vi "Insight_RW_Sweep_Profile.vi"(6 "String":string, 7 "Edge Roll-off (dB)":dbl=10.0 min=0.0 max=0.0, 8 "error in (no error)":errorcluster, 9 "Mode (Read / Write)":enum8{"Write", "Read"}(ring), 10 "Power Profile":enum16{"FLAT", "GAUSsian", "CUSTom"}(ring), 11 "telnet connection":T1) -> (0 "error out":errorcluster, 1 "response data":string, 2 "Power Profile":enum16{"FLAT", "GAUSsian", "CUSTom"}(ring), 3 "telnet  connection out":T1, 4 "Rolloff (dB)":dbl)   [LabVIEW 2015]
doc: "Insight Photonic Solutions\n\nThis VI reads or writes the sweep Power vs. Wavelength profile of the laser.\n\nINPUTS\n\nTelnet connection - reference to the Telnet connection\nMode - specifies if the command is a read or write\nPower Profile - specifies the type of commanded Power Profile\nEdge Roll-off - specifies the roll-off of the power profile at the minimum and maximum wavelengths of a Gaussian sweep in decibels down from the peak power value\nError In - the LabView error cluster, for tracking errors and enforcing sequentiality\n\nOUTPUTS\n\nTelnet Connection Out - reference out for the Telnet connection\nresponse data - string returned from the laser in response to a read or write\nPower Profile - Power Profile returned from the laser, parsed from the response data\nError Out - the LabView error cluster, for tracking errors and enforcing sequentiality\n\nREVISION HISTORY\nver 1.0 - original release\nver 1.1 - return the full response string and capture error if the parameter or command is not recognized.\nver 3.3 - modified to support earlier versions of this command (v3.2 and earlier), and current response format (3.3 and later)\nver 3.5 - modified to support new syntax of specifying the power profile and the rolloff in the same command for Gaussians"
uses:
  Telnet Session.ctl
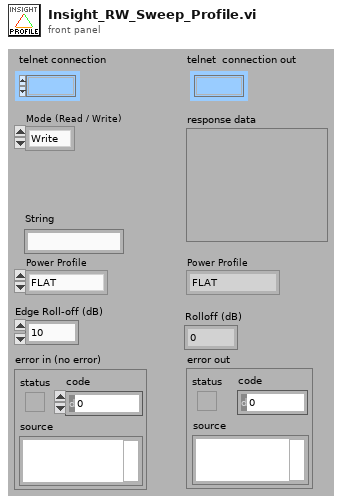
[diagram p1: front panel]
types:
  T1 = typedef "Telnet Session.ctl" = refnum<k1>
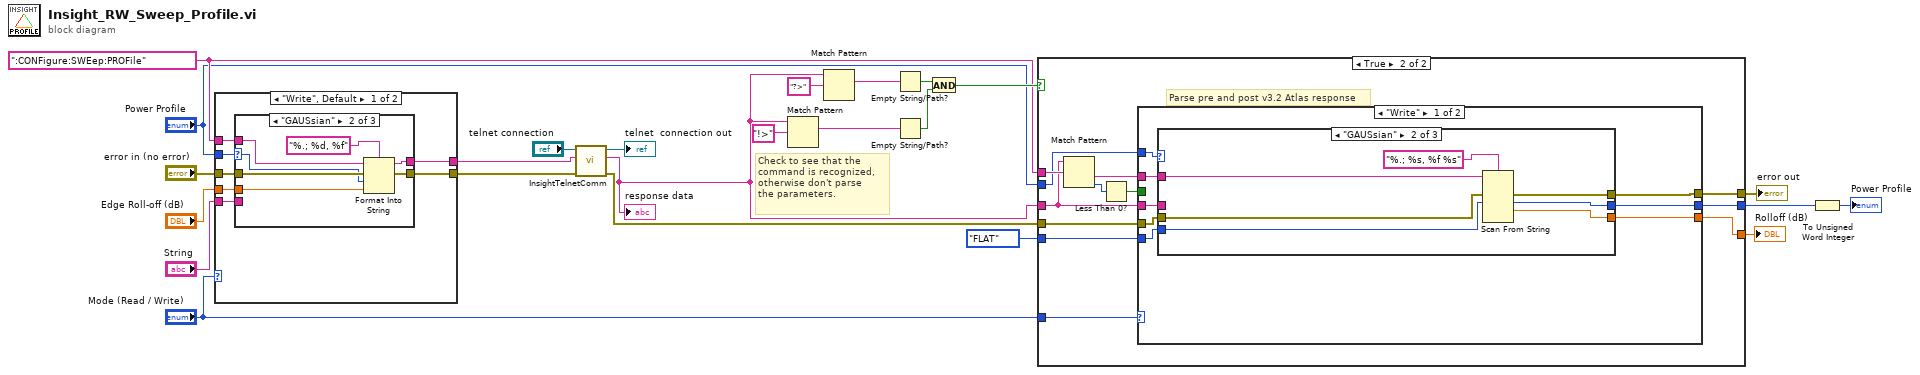
[diagram p0: block diagram]
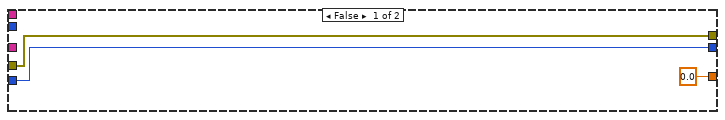
[diagram p2: hidden frame]
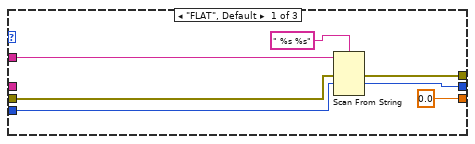
[diagram p3: hidden frame]
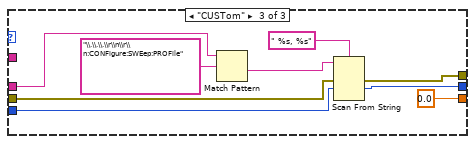
[diagram p4: hidden frame]
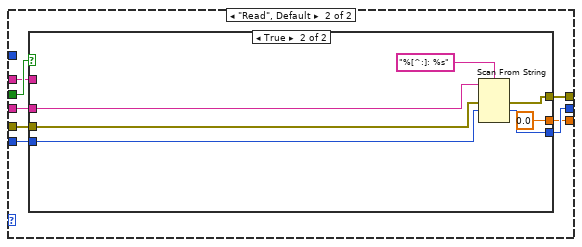
[diagram p5: hidden frame]
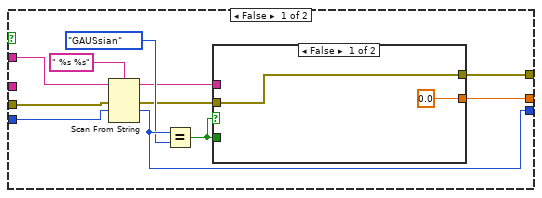
[diagram p6: hidden frame]
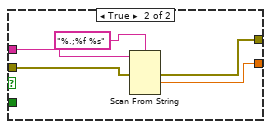
[diagram p7: hidden frame]
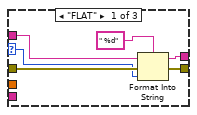
[diagram p8: hidden frame]
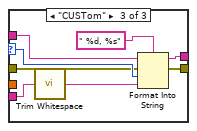
[diagram p9: hidden frame]
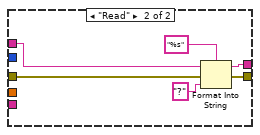
[diagram p10: hidden frame]
diagram:
  w12 = ":CONFigure:SWEep:PROFile" ("String")
  # "Check to see that the \ncommand is recognized,\notherwise don't parse \nthe parameters."
  n1 = case shown="\"Write\", Default" "Mode (Read / Write)" {
    tunnel: [w31 w54] -> w23
    tunnel: "error in (no error)" -> [w30 w53]
    tunnel: w12 -> [w29 w56]
    tunnel: [w28 w55] -> w22
    tunnel: "Power Profile" -> [w27 _]
    tunnel: "Edge Roll-off (dB)" -> [w26 _]
    tunnel: "String" -> [w25 _]
    frame "Write", Default {
      n2 = case shown="\"GAUSsian\"" w27 {
        selector: w27 -> [w32 w39 w51]
        tunnel: [w37 w44 w48] -> w31
        tunnel: w30 -> [w36 w43 w49]
        tunnel: w29 -> [w35 w42 w50]
        tunnel: [w33 w40 w47] -> w28
        tunnel: w26 -> [_ w38 _]
        tunnel: w25 -> [_ _ w46]
        frame "FLAT" {
          n3 = Format Into String(format string=" %d", initial string=w35, error in=w36, w32) -> (resulting string=w33:string, error out=w37:errorcluster)
        }
        frame "GAUSsian" {
          n4 = Format Into String(format string="%.; %d, %f", initial string=w42, error in=w43, w39, w38) -> (resulting string=w40:string, error out=w44:errorcluster)
        }
        frame "CUSTom" {
          n5 = call <vilib>:"Trim Whitespace.vi"("string"=w46) -> ("trimmed string"=w45:string)  [unwired: 1 in]
          n6 = Format Into String(format string=" %d, %s", initial string=w50, error in=w49, w51, w45) -> (resulting string=w47:string, error out=w48:errorcluster)
        }
      }
    }
    frame "Read" {
      n7 = Format Into String(format string="%s", initial string=w56, error in=w53, "?" ("input 1")) -> (resulting string=w55:string, error out=w54:errorcluster)
    }
  }
  n8 = call "InsightTelnetComm.vi"("error in"=w23, "write buffer (\"\")"=w22, "telnet connection"="telnet connection") -> ("error out"=w11:errorcluster, "response data"=w10:string, "telnet  connection out"=→"telnet  connection out":T1)  [unwired: 4 in]
  "response data" <- w10
  n9 = Match Pattern(string=w10, regular expression="!>") -> (match substring=w16:string)  [unwired: 1 in, 3 out]
  n10 = Match Pattern(string=w10, regular expression="?>") -> (match substring=w15:string)  [unwired: 1 in, 3 out]
  n11 = Empty String/Path?(string/path=w15) -> (empty?=w18:bool)
  n12 = Empty String/Path?(string/path=w16) -> (empty?=w19:bool)
  n13 = And(x=w18, y=w19) -> (x .and. y?=w13:bool)
  n14 = case shown="True" w13 {
    tunnel: w11 -> [w61 w67]
    tunnel: w10 -> [_ w64]
    tunnel: w12 -> [_ w72]
    tunnel: enum16{"FLAT", "GAUSsian", "CUSTom"}."FLAT" ("Power Profile") -> [w60 w68]
    tunnel: "Power Profile" -> [_ w63]
    tunnel: "Mode (Read / Write)" -> [_ w71]
    tunnel: [w61 w66] -> w3
    tunnel: [w60 w65] -> w2
    tunnel: [0.0 w62] -> w1
    frame False {
    }
    frame True {
      # "Parse pre and post v3.2 Atlas response"
      n15 = Match Pattern(string=w64, regular expression=w72) -> (after substring=w69:string, offset past match=w73:i32)  [unwired: 1 in, 2 out]
      n16 = Less Than 0?(x=w73) -> (x < 0?=w70:bool)
      n17 = case shown="\"Write\"" w71 {
        tunnel: w70 -> [_ w112]
        tunnel: w69 -> [w75 w111]
        tunnel: w68 -> [w80 w107]
        tunnel: w67 -> [w78 w110]
        tunnel: [w77 w109] -> w66
        tunnel: [w79 w108] -> w65
        tunnel: w64 -> [w81 w106]
        tunnel: w63 -> [w76 _]
        tunnel: [w74 w105] -> w62
        frame "Write" {
          n18 = case shown="\"GAUSsian\"" w76 {
            tunnel: [w87 w91 w103] -> w79
            tunnel: w81 -> [_ _ w101]
            tunnel: w80 -> [w86 w92 w99]
            tunnel: w78 -> [w85 w93 w98]
            tunnel: [w84 w90 w97] -> w77
            tunnel: w75 -> [w83 w94 _]
            tunnel: [0.0 w89 0.0] -> w74
            frame "FLAT", Default {
              n19 = Scan From String(format string=" %s %s", input string=w83, error in=w85, default 1=w86) -> (error out=w84:errorcluster, output 1=w87:enum16{"FLAT", "GAUSsian", "CUSTom"})  [unwired: 3 in, 2 out]
            }
            frame "GAUSsian" {
              n20 = Scan From String(format string="%.; %s, %f %s" ("f"), input string=w94, error in=w93, default 1=w92) -> (error out=w90:errorcluster, output 1=w91:enum16{"FLAT", "GAUSsian", "CUSTom"}, output 2=w89:dbl)  [unwired: 4 in, 2 out]
            }
            frame "CUSTom" {
              n21 = Match Pattern(string=w101, regular expression="\\.\\.\\.\\r\\n\\r\\n:CONFigure:SWEep:PROFile") -> (after substring=w100:string)  [unwired: 1 in, 3 out]
              n22 = Scan From String(format string=" %s, %s" ("f"), input string=w100, error in=w98, default 1=w99) -> (error out=w97:errorcluster, output 1=w103:enum16{"FLAT", "GAUSsian", "CUSTom"})  [unwired: 3 in, 2 out]
            }
          }
        }
        frame "Read", Default {
          n23 = case shown="True" w112 {
            tunnel: w111 -> [w122 _]
            tunnel: w110 -> [w121 w136]
            tunnel: [w113 w133] -> w109
            tunnel: [w119 w134] -> w108
            tunnel: w107 -> [w120 w135]
            tunnel: w106 -> [_ w132]
            tunnel: [w115 0.0] -> w105
            frame False {
              n24 = Scan From String(format string=" %s %s" ("f"), input string=w122, error in=w121, default 1=w120) -> (remaining string=w116:string, error out=w114:errorcluster, output 1=w119:enum16{"FLAT", "GAUSsian", "CUSTom"})  [unwired: 3 in, 1 out]
              n25 = Equal?(x=w119, y=enum16{"FLAT", "GAUSsian", "CUSTom"}."GAUSsian") -> (x = y?=w117:bool)
              n26 = case shown="False" w117 {
                tunnel: w117 -> [_ _]
                tunnel: w116 -> [_ w130]
                tunnel: [0.0 w128] -> w115
                tunnel: w114 -> [w125 w127]
                tunnel: [w125 w126] -> w113
                frame False {
                }
                frame True {
                  n27 = Scan From String(format string="%.;%f %s", input string=w130, error in=w127) -> (error out=w126:errorcluster, output 1=w128:dbl)  [unwired: 4 in, 2 out]
                }
              }
            }
            frame True {
              n28 = Scan From String(format string="%[^:]: %s", input string=w132, error in=w136, default 1=w135) -> (error out=w133:errorcluster, output 1=w134:enum16{"FLAT", "GAUSsian", "CUSTom"})  [unwired: 3 in, 2 out]
            }
          }
        }
      }
    }
  }
  "error out" <- w3
  "Rolloff (dB)" <- w1
  n29 = To Unsigned Word Integer(number=w2) -> (unsigned 16bit integer=→"Power Profile":u16)
